vi "DRAW FP PAQUETES IN UI.vi"(8 "error in (no error)":errorcluster, 11 "Paquetes in":refnum<class "Paquetes.lvclass">) -> (0 "error out":errorcluster, 3 "Paquetes out":refnum<class "Paquetes.lvclass">)   [LabVIEW 2020, in "Paquetes.lvlib" / "Paquetes.lvclass"]
uses:
  Paquetes.lvclass
  Paquetes.lvclass/Paquetes.ctl
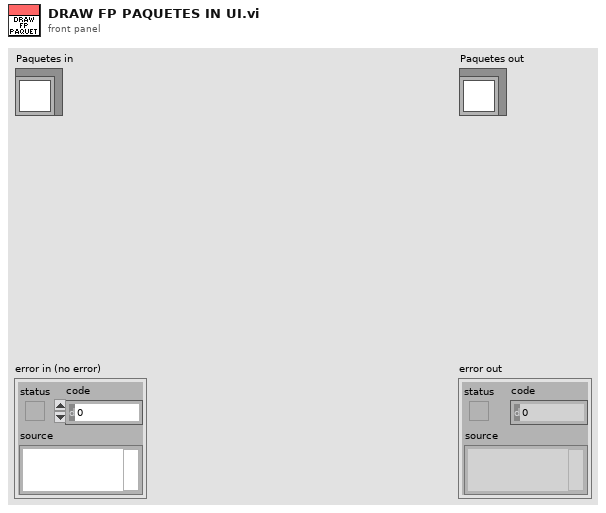
[diagram p1: front panel]
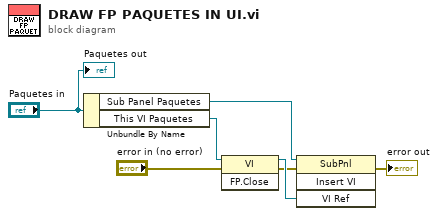
[diagram p0: block diagram]
diagram:
  n1 = Unbundle By Name("Paquetes in") -> ("Sub Panel Paquetes"=w3:refnum<vi>, "This VI Paquetes"=w6:refnum<vi>)
  n2 = invoke class="VI" method="FP.Close"(reference=w6, error in="error in (no error)") -> (reference out=w7:refnum<vi>, error out=w5:errorcluster)  [unwired: 1 in, 1 out]
  n3 = invoke class="SubPnl" method="Insert VI"(reference=w3, error in=w5, "VI Ref"=w7) -> (error out=→"error out":errorcluster)  [unwired: 1 in, 3 out]
  "Paquetes out" <- "Paquetes in"
